vi "Halvorsen_1D_Lyapunov.vi"(11 "Initial Conditions":ext[](array[numeric])=[0.150000000000000000005, 0.1, 0.1]) -> ()   [LabVIEW 2016]
panel:
  in  "Initial Conditions Inc.":ext[](array[numeric])=[1e-8, 1e-8, 1e-8]
  in  "Tab Control":T1(tab)
  out "Mode Analysis":cluster{ext[], dbl[]}[](graph)=[{array[380 elements], [21.0, 25.0, 13.0, 26.0, 10.0, 21.0, 27.0, 22.0, 5.0, 15.0, 19.0, 19.0, 14.0, 15.0, 28.0, 21.0, 17.0, 26.0, 16.0, 16.0, 21.0, 21.0, 18.0, 1.0, 10.0, 13.0, 12.0, 14.0, 13.0, 12.0, 10.0, 16.0, 1.0, 10.0, 2.0, 16.0, 21.0, 4.0, 24.0, 20.0, 18.0, 14.0, 8.0, 23.0, 20.0, 11.0, 16.0, 26.0, 23.0, 25.0, 7.0, 16.0, 14.0, 17.0, 23.0, 13.0, 6.0, 21.0, 27.0, 24.0, 9.0, 7.0, 11.0, 19.0, 10.0, 17.0, 14.0, 8.0, 12.0, 16.0, 19.0, 19.0, 20.0, 16.0, 17.0, 22.0, 16.0, 18.0, 21.0, 27.0, 19.0, 23.0, 22.0, 19.0, 18.0, 17.0, 18.0, 13.0, 23.0, 14.0, 14.0, 19.0, 15.0, 22.0, 6.0, 16.0, 25.0, 18.0, 23.0, 18.0, 24.0, 22.0, 22.0, 20.0, 23.0, 21.0, 21.0, 19.0, 29.0, 18.0, 22.0, 16.0, 11.0, 16.0, 18.0, 18.0, 26.0, 24.0, 27.0, 28.0, 24.0, 21.0, 15.0, 24.0, 18.0, 19.0, 18.0, 23.0, 12.0, 20.0, 14.0, 17.0, 21.0, 24.0, 27.0, 27.0, 23.0, 19.0, 7.0, 24.0, 15.0, 24.0, 27.0, 19.0, 21.0, 21.0, 20.0, 16.0, 26.0, 21.0, 24.0, 24.0, 30.0, 19.0, 10.0, 18.0, 23.0, 25.0, 25.0, 20.0, 21.0, 21.0, 19.0, 24.0, 14.0, 18.0, 16.0, 21.0, 22.0, 20.0, 16.0, 24.0, 21.0, 24.0, 20.0, 20.0, 20.0, 24.0, 21.0, 22.0, 18.0, 27.0, 18.0, 21.0, 21.0, 18.0, 22.0, 20.0, 21.0, 21.0, 22.0, 19.0, 19.0, 15.0, 19.0, 19.0, 21.0, 18.0, 10.0, 20.0, 21.0, 20.0, 20.0, 18.0, 13.0, 20.0, 23.0, 18.0, 20.0, 17.0, 21.0, 20.0, 8.0, 5.0, 5.0, 19.0, 5.0, 16.0, 15.0, 5.0, 13.0, 19.0, 17.0, 17.0, 19.0, 13.0, 18.0, 19.0, 19.0, 20.0, 17.0, 16.0, 14.0, 16.0, 17.0, 15.0, 14.0, 15.0, 8.0, 17.0, 4.0, 17.0, 15.0, 17.0, 17.0, 16.0, 20.0, 17.0, 11.0, 7.0, 6.0, 11.0, 18.0, 8.0, 8.0, 18.0, 9.0, 16.0, 16.0, 19.0, 18.0, 15.0, 17.0, 16.0, 13.0, 13.0, 6.0, 5.0, 5.0, 4.0, 4.0, 4.0, 6.0, 19.0, 17.0, 8.0, 14.0, 15.0, 14.0, 17.0, 17.0, 10.0, 18.0, 11.0, 17.0, 12.0, 17.0, 2.0, 2.0, 1.0, 1.0, 2.0, 2.0, 2.0, 2.0, 2.0, 2.0, 2.0, 2.0, 2.0, 2.0, 2.0, 2.0, 2.0, 2.0, 2.0, 2.0, 4.0, 2.0, 17.0, 5.0, 4.0, 5.0, 8.0, 10.0, 12.0, 13.0, 13.0, 11.0, 9.0, 7.0, 2.0, 2.0, 2.0, 2.0, 2.0, 2.0, 2.0, 2.0, 2.0, 1.0, 2.0, 2.0, 2.0, 2.0, 2.0, 2.0, 2.0, 2.0, 2.0, 2.0, 2.0, 2.0, 2.0, 2.0, 2.0, 2.0, 2.0, 2.0, 2.0, 2.0, 1.0, 2.0, 5.0, 15.0, 12.0, 22.0, 13.0, 13.0, 9.0, 18.0, 10.0, 19.0, 17.0, 23.0, 23.0, 9.0, 7.0, 18.0, 21.0, 20.0, 19.0, 20.0, 20.0, 20.0, 9.0, 19.0, 18.0, 23.0, 17.0]}, {array[380 elements], [22.0, 26.0, 14.0, 26.0, 11.0, 21.0, 28.0, 23.0, 6.0, 16.0, 20.0, 20.0, 15.0, 16.0, 29.0, 21.0, 17.0, 26.0, 17.0, 17.0, 22.0, 22.0, 19.0, 1.0, 11.0, 14.0, 12.0, 15.0, 14.0, 13.0, 11.0, 17.0, 0.0, 10.0, 3.0, 17.0, 22.0, 5.0, 24.0, 20.0, 19.0, 15.0, 9.0, 23.0, 21.0, 12.0, 16.0, 27.0, 24.0, 25.0, 7.0, 17.0, 15.0, 18.0, 24.0, 14.0, 7.0, 22.0, 25.0, 25.0, 10.0, 8.0, 12.0, 20.0, 11.0, 17.0, 15.0, 8.0, 13.0, 17.0, 19.0, 19.0, 21.0, 17.0, 18.0, 22.0, 17.0, 18.0, 19.0, 26.0, 17.0, 23.0, 22.0, 19.0, 18.0, 17.0, 18.0, 13.0, 24.0, 14.0, 10.0, 20.0, 16.0, 22.0, 7.0, 17.0, 24.0, 13.0, 21.0, 17.0, 24.0, 19.0, 21.0, 20.0, 22.0, 21.0, 21.0, 20.0, 30.0, 19.0, 20.0, 16.0, 10.0, 15.0, 16.0, 18.0, 24.0, 24.0, 25.0, 27.0, 24.0, 22.0, 16.0, 25.0, 18.0, 20.0, 18.0, 23.0, 12.0, 20.0, 15.0, 9.0, 21.0, 24.0, 25.0, 25.0, 22.0, 17.0, 5.0, 25.0, 15.0, 23.0, 26.0, 18.0, 22.0, 21.0, 20.0, 15.0, 26.0, 19.0, 22.0, 25.0, 27.0, 19.0, 10.0, 18.0, 24.0, 26.0, 22.0, 20.0, 21.0, 21.0, 18.0, 24.0, 13.0, 19.0, 15.0, 21.0, 22.0, 16.0, 17.0, 22.0, 22.0, 22.0, 19.0, 19.0, 19.0, 19.0, 21.0, 23.0, 18.0, 26.0, 19.0, 20.0, 21.0, 18.0, 18.0, 21.0, 19.0, 21.0, 20.0, 16.0, 18.0, 13.0, 13.0, 19.0, 21.0, 14.0, 5.0, 19.0, 21.0, 20.0, 19.0, 19.0, 8.0, 19.0, 20.0, 17.0, 20.0, 14.0, 18.0, 17.0, 6.0, 5.0, 6.0, 18.0, 5.0, 15.0, 10.0, 4.0, 10.0, 16.0, 16.0, 17.0, 19.0, 14.0, 19.0, 18.0, 19.0, 18.0, 15.0, 13.0, 12.0, 17.0, 16.0, 15.0, 13.0, 12.0, 7.0, 18.0, 4.0, 15.0, 16.0, 14.0, 17.0, 16.0, 19.0, 12.0, 7.0, 6.0, 4.0, 6.0, 16.0, 8.0, 7.0, 19.0, 8.0, 14.0, 17.0, 16.0, 19.0, 13.0, 17.0, 13.0, 11.0, 12.0, 5.0, 4.0, 4.0, 4.0, 4.0, 4.0, 4.0, 19.0, 17.0, 8.0, 13.0, 14.0, 10.0, 16.0, 14.0, 11.0, 15.0, 11.0, 14.0, 13.0, 15.0, 2.0, 2.0, 1.0, 1.0, 2.0, 2.0, 2.0, 2.0, 2.0, 2.0, 2.0, 2.0, 2.0, 2.0, 2.0, 2.0, 2.0, 2.0, 2.0, 2.0, 2.0, 2.0, 9.0, 4.0, 4.0, 4.0, 4.0, 4.0, 4.0, 4.0, 3.0, 2.0, 2.0, 2.0, 2.0, 2.0, 2.0, 2.0, 2.0, 2.0, 2.0, 2.0, 2.0, 1.0, 2.0, 2.0, 2.0, 2.0, 2.0, 2.0, 2.0, 2.0, 2.0, 2.0, 2.0, 2.0, 2.0, 2.0, 2.0, 2.0, 2.0, 2.0, 2.0, 2.0, 1.0, 2.0, 2.0, 15.0, 10.0, 15.0, 12.0, 10.0, 8.0, 12.0, 9.0, 14.0, 13.0, 14.0, 13.0, 6.0, 6.0, 12.0, 12.0, 14.0, 16.0, 15.0, 15.0, 13.0, 8.0, 15.0, 13.0, 16.0, 11.0]}]
  out "Waveform Graph":ext[][](graph)
  out "?":cluster{ext[], ext[]}[](graph)
  out "Bifurcation Diagram":cluster{ext[], ext[]}(graph)
  in  "Parameter Index":i32
  in  "Final Parameter Value":dbl=0.2
  in  "Param_Inc":dbl[](array[numeric])=[0.0005, 0.0, 0.0]
  in  "Initial_Parameter_Vector":ext[](array[numeric])=[0.01, 0.1, 0.1]
  out "Current_Param":ext[](array[numeric])=[0.20000000000000000395, 0.1, 0.1]
  in  "Variable":u16(ring) items=["x", "y", "z"]
  in  "Время, с":ext=500.0
  in  "Hmin":ext=0.00099999999999999999996
  in  "Hmax":ext=1.0
  in  "tolerance":ext=1e-13
  in  "Шаг h, с":ext=0.01
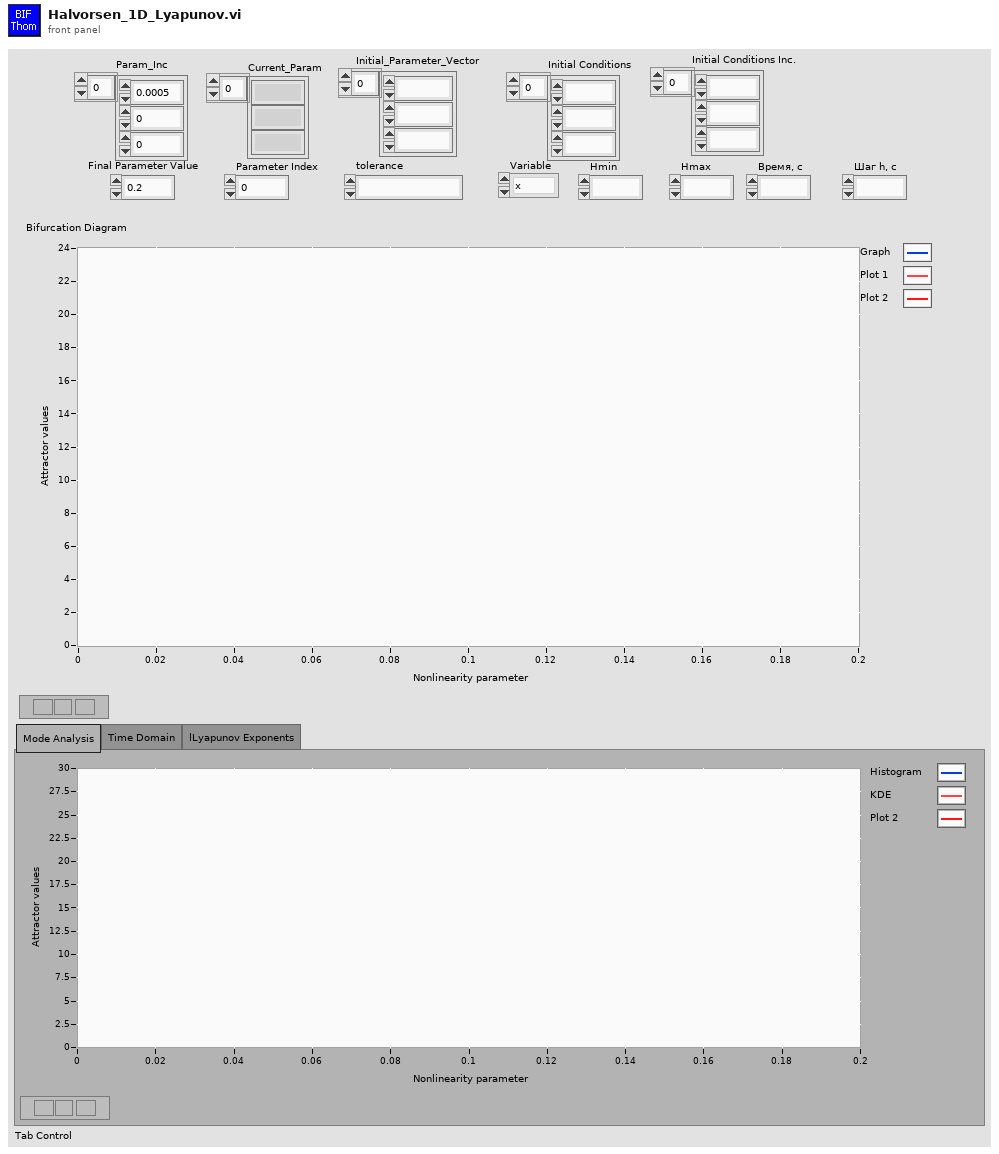
[diagram p1: front panel]
types:
  T1 = enum32{"Mode Analysis", "Time Domain", "lLyapunov Exponents"}
  T2 = enum16{"Euler", "Cromer 1", "Cromer 2", "D1", "D2", "PD1", "PD2", "CD1", "CD2", "CD3", "CD4", "IMP", "LIMP", "IEuler", "SEMP", "SIMP", "EMP", "MEMP"}
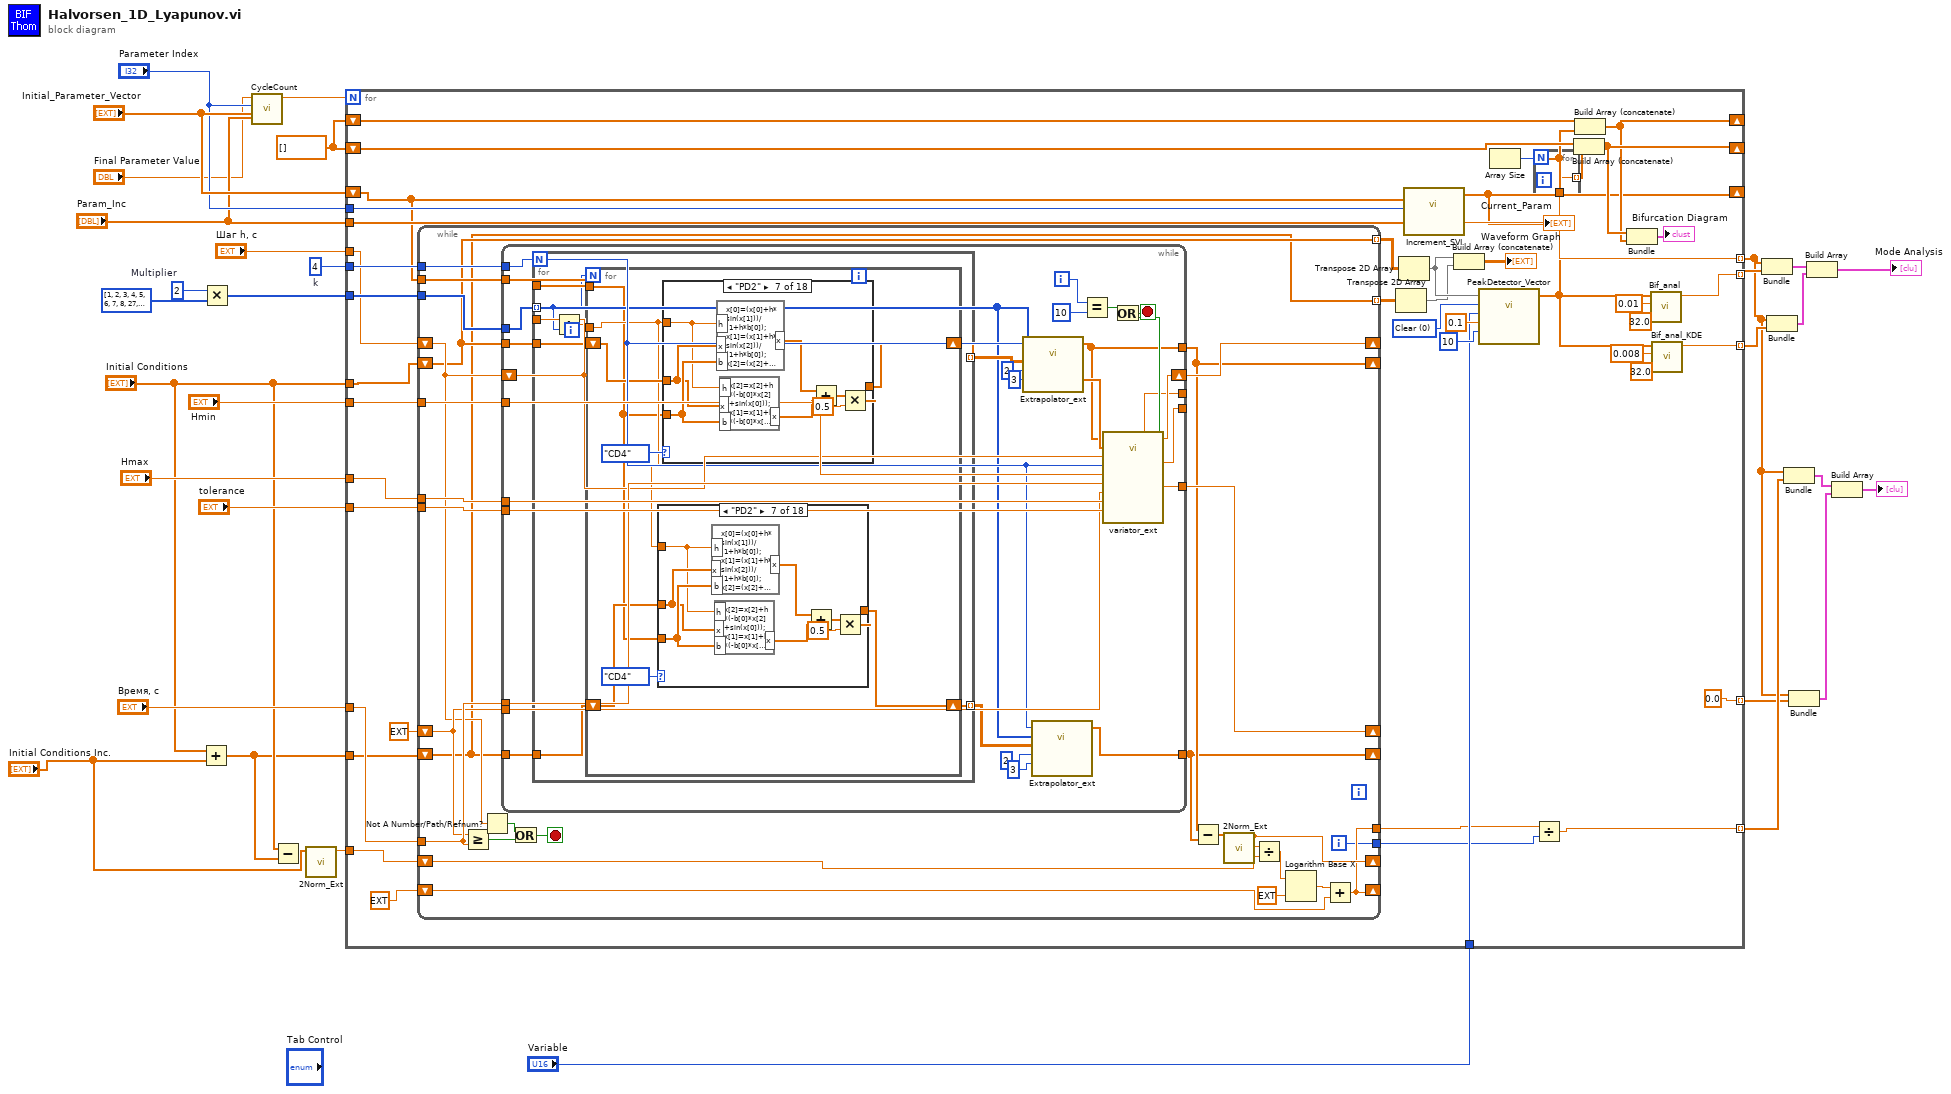
[diagram p0: block diagram]
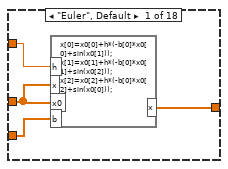
[diagram p2: hidden frame]
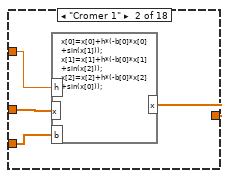
[diagram p3: hidden frame]
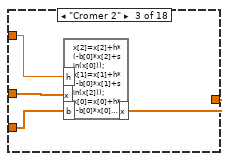
[diagram p4: hidden frame]
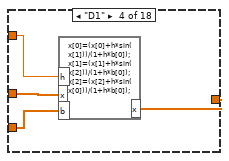
[diagram p5: hidden frame]
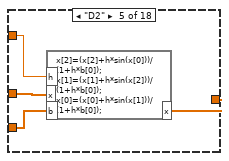
[diagram p6: hidden frame]
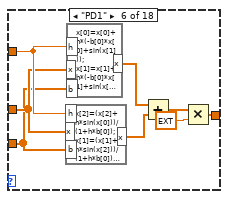
[diagram p7: hidden frame]
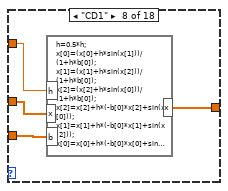
[diagram p8: hidden frame]
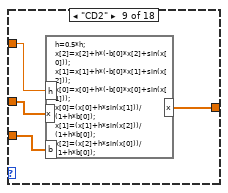
[diagram p9: hidden frame]
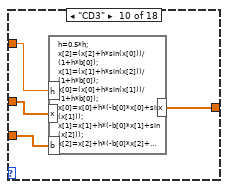
[diagram p10: hidden frame]
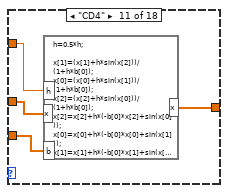
[diagram p11: hidden frame]
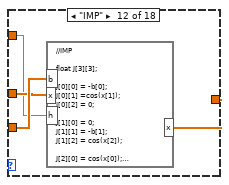
[diagram p12: hidden frame]
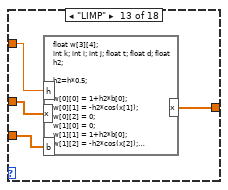
[diagram p13: hidden frame]
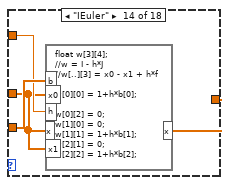
[diagram p14: hidden frame]
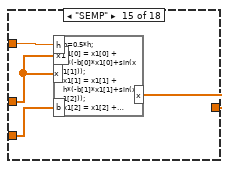
[diagram p15: hidden frame]
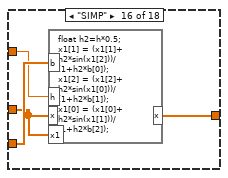
[diagram p16: hidden frame]
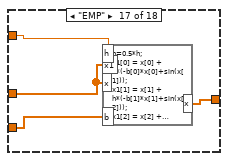
[diagram p17: hidden frame]
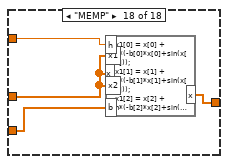
[diagram p18: hidden frame]
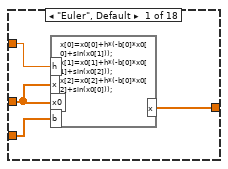
[diagram p19: hidden frame]
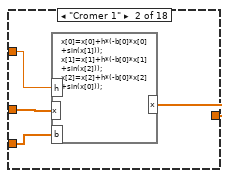
[diagram p20: hidden frame]
diagram:
  w16 = ext[] []
  w18 = 4  # k
  w21 = 2  # Multiplier
  n1 = Add(x="Initial Conditions", y="Initial Conditions Inc.") -> (x+y=w9:ext[])
  n2 = Multiply(x=w21, y=i32[] [1, 2, 3, 4, 5, 6, 7, 8, 27, 30, 33] ("n")) -> (x*y=w19:i32[])
  n3 = call "CycleCount.vi"("Increment_Vector"="Param_Inc", "Parameter_Vector"="Initial_Parameter_Vector", "Parameter Number"="Parameter Index", "Final_Parameter_Value"="Final Parameter Value") -> ("Cycle Count"=w17:ext)  [unwired: 5 in, 2 out]
  n4 = Subtract(x="Initial Conditions", y=w9) -> ()  [unwired: 1 out]
  n5 = call "2Norm_Ext.vi"("Input vector"="Initial Conditions Inc.") -> ("2 Norm"=w8:ext)  [unwired: 10 in]
  n6 = for {
    N: w17 -> [_]
    tunnel: w18 -> [w52]
    tunnel: "Шаг h, с" -> [w43]
    tunnel: "Время, с" -> [w47]
    tunnel: "tolerance" -> [w45]
    tunnel: "Hmin" -> [w49]
    tunnel: "Hmax" -> [w48]
    tunnel: w19 -> [w44]
    tunnel: "Initial Conditions" -> [w50]
    shift-right: [w54] -> _
    shift-left: "Initial_Parameter_Vector" -> [w51]
    tunnel: "Parameter Index" -> [w72]
    tunnel: "Param_Inc" -> [w71]
    tunnel: [w70] -> w15 mode=indexing
    tunnel: "Variable" -> [w69]
    shift-right: [w62] -> _
    shift-left: w16 -> [w67]
    shift-right: [w63] -> _
    shift-left: w16 -> [w66]
    tunnel: [w61] -> w6 mode=indexing
    tunnel: [w55] -> w12 mode=indexing
    tunnel: w9 -> [w42]
    tunnel: w8 -> [w40]
    tunnel: [w34] -> w7 mode=indexing
    tunnel: [0.0] -> w5 mode=indexing
    w75 = u16 0 items=["Clear", "Absolute", "Positive"] ("Signal Mode")
    n7 = while {
      shift-right: [w82] -> _
      shift-left: w50 -> [w88]
      tunnel: w44 -> [w102]
      tunnel: w52 -> [w101]
      shift-right: [w97] -> _
      shift-left: w43 -> [w90]
      shift-right: [w94] -> _
      shift-left: ext 0.0 ("New time") -> [w95]
      tunnel: w47 -> [w96]
      tunnel: w45 -> [w98]
      tunnel: w49 -> [w100]
      tunnel: w48 -> [w99]
      tunnel: w51 -> [w93]
      tunnel: [w88] -> w53 mode=indexing
      shift-right: [w81] -> _
      shift-left: w42 -> [w78]
      shift-right: [w79] -> _
      shift-left: w40 -> [w83]
      shift-right: [w77] -> _
      shift-left: ext 0.0 -> [w84]
      tunnel: [w78] -> w39 mode=indexing
      tunnel: [w77] -> w33
      tunnel: [w76] -> w32
      i -> [w76]
      stop <- w92 stop-if-true
      n8 = Greater Or Equal?(x=w95, y=w96) -> (x >= y?=w91:bool)
      n9 = Not A Number/Path/Refnum?(number/path/refnum=w90) -> (NaN/Path/Refnum?=w89:bool)
      n10 = while {
        tunnel: w100 -> [w125]
        tunnel: w99 -> [w128]
        tunnel: w98 -> [w124]
        tunnel: w101 -> [w108]
        tunnel: w102 -> [w107]
        tunnel: w88 -> [w126]
        shift-right: [w119] -> w97
        shift-left: w90 -> [w111]
        tunnel: [w111] -> _
        tunnel: [w118] -> _
        tunnel: [w117] -> w82
        tunnel: w96 -> [w116]
        tunnel: w95 -> [w115]
        tunnel: [w113] -> w94
        tunnel: w93 -> [w112]
        tunnel: w78 -> [w109]
        tunnel: [w103] -> w81
        i -> [w114]
        stop <- w120 stop-if-true
        n11 = for {
          N: w108 -> [_]
          tunnel: w107 -> [w133] mode=indexing
          tunnel: w111 -> [w138]
          tunnel: w126 -> [w136]
          tunnel: [w137] -> w127 mode=indexing
          tunnel: w112 -> [w134]
          tunnel: w109 -> [w132]
          tunnel: [w131] -> w106 mode=indexing
          n12 = Divide(x=w138, y=w133) -> (x/y=w135:ext)
          n13 = for {
            N: w133 -> [_]
            shift-right: [w146] -> w137
            shift-left: w136 -> [w145]
            tunnel: w135 -> [w142]
            tunnel: w134 -> [w139]
            shift-right: [w140] -> w131
            shift-left: w132 -> [w141]
            n14 = case shown="\"PD2\"" T2."CD4" ("Method") {
              tunnel: w142 -> [w148 w154 w157 w161 w166 w169 w175 w185 w189 w194 w197 w199 w206 w209 w213 w216 w220 w224]
              tunnel: w139 -> [w150 w152 w155 w159 w164 w167 w177 w183 w187 w192 w195 w201 w203 w210 w211 w217 w221 w225]
              tunnel: w141 -> [w149 w153 w156 w160 w165 w168 w176 w184 w188 w193 w196 w200 w204 w208 w212 w215 w219 w226]
              tunnel: [w147 w151 w158 w162 w163 w170 w178 w186 w190 w191 w198 w202 w205 w207 w214 w218 w222 w223] -> w140
              frame "Euler", Default {
                n15 = formula code="x[0]=x0[0]+h*(-b[0]*x0[0]+sin(x0[1]));\nx[1]=x0[1]+h*(-b[0]*x0[1]+sin(x0[2]));\nx[2]=x0[2]+h*(-b[0]*x0[2]+sin(x0[0]));"("x"=w149, "x0"=w149, "b"=w150, "h"=w148) -> ("x"=w147:ext[])
              }
              frame "Cromer 1" {
                n16 = formula code="x[0]=x[0]+h*(-b[0]*x[0]+sin(x[1]));\nx[1]=x[1]+h*(-b[0]*x[1]+sin(x[2]));\nx[2]=x[2]+h*(-b[0]*x[2]+sin(x[0]));"("x"=w153, "b"=w152, "h"=w154) -> ("x"=w151:ext[])
              }
              frame "Cromer 2" {
                n17 = formula code="x[2]=x[2]+h*(-b[0]*x[2]+sin(x[0]));\nx[1]=x[1]+h*(-b[0]*x[1]+sin(x[2]));\nx[0]=x[0]+h*(-b[0]*x[0]+sin(x[1]));"("x"=w156, "b"=w155, "h"=w157) -> ("x"=w158:ext[])
              }
              frame "D1" {
                n18 = formula code="x[0]=(x[0]+h*sin(x[1]))/(1+h*b[0]);\nx[1]=(x[1]+h*sin(x[2]))/(1+h*b[0]);\nx[2]=(x[2]+h*sin(x[0]))/(1+h*b[0]);"("x"=w160, "b"=w159, "h"=w161) -> ("x"=w162:ext[])
              }
              frame "D2" {
                n19 = formula code="x[2]=(x[2]+h*sin(x[0]))/(1+h*b[0]);\nx[1]=(x[1]+h*sin(x[2]))/(1+h*b[0]);\nx[0]=(x[0]+h*sin(x[1]))/(1+h*b[0]);"("x"=w165, "b"=w164, "h"=w166) -> ("x"=w163:ext[])
              }
              frame "PD1" {
                n20 = formula code="x[2]=(x[2]+h*sin(x[0]))/(1+h*b[0]);\nx[1]=(x[1]+h*sin(x[2]))/(1+h*b[0]);\nx[0]=(x[0]+h*sin(x[1]))/(1+h*b[0]);"("x"=w168, "b"=w167, "h"=w169) -> ("x"=w172:ext[])
                n21 = formula code="x[0]=x[0]+h*(-b[0]*x[0]+sin(x[1]));\nx[1]=x[1]+h*(-b[0]*x[1]+sin(x[2]));\nx[2]=x[2]+h*(-b[0]*x[2]+sin(x[0]));"("x"=w168, "b"=w167, "h"=w169) -> ("x"=w171:ext[])
                n22 = Add(x=w171, y=w172) -> (x+y=w173:ext[])
                n23 = Multiply(x=w173, y=ext 0.5) -> (x*y=w170:ext[])
              }
              frame "PD2" {
                n24 = formula code="x[0]=(x[0]+h*sin(x[1]))/(1+h*b[0]);\nx[1]=(x[1]+h*sin(x[2]))/(1+h*b[0]);\nx[2]=(x[2]+h*sin(x[0]))/(1+h*b[0]);"("x"=w176, "b"=w177, "h"=w175) -> ("x"=w182:ext[])
                n25 = formula code="x[2]=x[2]+h*(-b[0]*x[2]+sin(x[0]));\nx[1]=x[1]+h*(-b[0]*x[1]+sin(x[2]));\nx[0]=x[0]+h*(-b[0]*x[0]+sin(x[1]));"("x"=w176, "b"=w177, "h"=w175) -> ("x"=w181:ext[])
                n26 = Add(x=w182, y=w181) -> (x+y=w180:ext[])
                n27 = Multiply(x=w180, y=0.5) -> (x*y=w178:ext[])
              }
              frame "CD1" {
                n28 = formula code="h=0.5*h;\nx[0]=(x[0]+h*sin(x[1]))/(1+h*b[0]);\nx[1]=(x[1]+h*sin(x[2]))/(1+h*b[0]);\nx[2]=(x[2]+h*sin(x[0]))/(1+h*b[0]);\nx[2]=x[2]+h*(-b[0]*x[2]+sin(x[0]));\nx[1]=x[1]+h*(-b[0]*x[1]+sin(x[2]));\nx[0]=x[0]+h*(-b[0]*x[0]+sin(x[1]));"("x"=w184, "b"=w183, "h"=w185) -> ("x"=w186:ext[])
              }
              frame "CD2" {
                n29 = formula code="h=0.5*h;\nx[2]=x[2]+h*(-b[0]*x[2]+sin(x[0]));\nx[1]=x[1]+h*(-b[0]*x[1]+sin(x[2]));\nx[0]=x[0]+h*(-b[0]*x[0]+sin(x[1]));\nx[0]=(x[0]+h*sin(x[1]))/(1+h*b[0]);\nx[1]=(x[1]+h*sin(x[2]))/(1+h*b[0]);\nx[2]=(x[2]+h*sin(x[0]))/(1+h*b[0]);"("x"=w188, "b"=w187, "h"=w189) -> ("x"=w190:ext[])
              }
              frame "CD3" {
                n30 = formula code="h=0.5*h;\nx[2]=(x[2]+h*sin(x[0]))/(1+h*b[0]);\nx[1]=(x[1]+h*sin(x[2]))/(1+h*b[0]);\nx[0]=(x[0]+h*sin(x[1]))/(1+h*b[0]);\nx[0]=x[0]+h*(-b[0]*x[0]+sin(x[1]));\nx[1]=x[1]+h*(-b[0]*x[1]+sin(x[2]));\nx[2]=x[2]+h*(-b[0]*x[2]+sin(x[0]));"("x"=w193, "b"=w192, "h"=w194) -> ("x"=w191:ext[])
              }
              frame "CD4" {
                n31 = formula code="h=0.5*h;\n\nx[1]=(x[1]+h*sin(x[2]))/(1+h*b[0]);\nx[0]=(x[0]+h*sin(x[1]))/(1+h*b[0]);\nx[2]=(x[2]+h*sin(x[0]))/(1+h*b[0]);\nx[2]=x[2]+h*(-b[0]*x[2]+sin(x[0]));\nx[0]=x[0]+h*(-b[0]*x[0]+sin(x[1]));\nx[1]=x[1]+h*(-b[0]*x[1]+sin(x[2]));"("x"=w196, "b"=w195, "h"=w197) -> ("x"=w198:ext[])
              }
              frame "IMP" {
                n32 = formula code="//IMP\n\nfloat J[3][3];\n\nJ[0][0] = -b[0]; \nJ[0][1] =cos(x[1]); \nJ[0][2] = 0; \n\nJ[1][0] = 0; \nJ[1][1] = -b[1];\nJ[1][2] = cos(x[2]);\n\nJ[2][0] = cos(x[0]); \nJ[2][1] =0;\nJ[2][2] = -b[2];\n\n\nfloat w[3][4], Z[3], a[3], Zn[3], dz;\nfloat tol;\nint k; int i; int j; float t; float d;\ntol = 1e-14;\nint nnewtmax = 3, nnewt;\ndz = 2e-13;\nnnewt = 0;\n\nZ[0] = x[0]; Z[1] = x[1]; Z[2] = x[2];\nwhile ( (dz > tol) && (nnewt < nnewtmax)){\n\nfor(i=0;i<3;i++){\nfor(j=0;j<3;j++){\nif (i==j)\nw[i][j]=1 - 0.5*h*J[i][j];\nelse\nw[i][j]= - 0.5*h*J[i][j];\n}}\n\n\n\na[0] = 0.5*(x[0] + Z[0]);\na[1] = 0.5*(x[1] + Z[1]);\na[2] = 0.5*(x[2] + Z[2]);\n\n\n\nw[0][3]=-Z[0]+x[0]+h*(-b[0]*a[0]+sin(a[1]));\nw[1][3]= -Z[1]+x[1]+h*(-b[1]*a[1]+sin(a[2]));\nw[2][3]= -Z[2]+x[2]+h*(-b[2]*a[2]+sin(a[0]));\n\n\nfor(k = 0; k <= 1; k++){\n\tint l = k;\n\n\tfor( i = k+1; i<= 2; i++){\n\t\tif( abs(w[i][k]) > abs(w[l][k]) ){\n\t\t\tl = i;\n\t\t}\n\t}\n\tif (l != k){\n\t\tfor( j = 0; j <= 3; j++){\n\t\t\tif ((j == 0) || (j >= k)){\n\t\t\t\tt = w[k][j];\n\t\t\t\tw[k][j] = w[l][j];\n\t\t\t\tw[l][j] = t;\n\t\t\t}\n\t\t}\n\t}\t\n\n\td = 1.0 / w[k][k];\n\tfor( i=(k+1); i <=(2); i++){\n\t\tif (w[i][k] == 0){\n\t\t\tcontinue;\n\t\t}\n\t\tt = w[i][k] * d;\n\t\tfor ( j = k; j <= (3); j++) {\n\t\t\tif (w[k][j] != 0){\n\t\t\t\tw[i][j] = w[i][j] - t * w[k][j];\n\t\t\t}\n\t\t}\n\t}\n}\nfor( i=(3); i >= 2; i--){\n\tfor( j=1; j <= i-1; j++){\n\t\tt = w[i - j - 1][i - 1]/w[ i -1][i - 1];\n\t\tw[i-j - 1][ 3] = w[i-j -1][3] - t*w[i - 1][ 3];\n\t}\n\tw[i-1][ 3] = w[i - 1][3]/w[ i -1][i - 1];\n}\nw[0][3] = w[0][3]/w[0][0];\nZn[0] = Z[0]+ w[0][3];\nZn[1] = Z[1]+ w[1][3];\nZn[2] = Z[2]+ w[2][3];\n\ndz = ( (Zn[0] - Z[0])**2 + (Zn[1] - Z[1])**2 + (Zn[2] - Z[2])**2 )**0.5;\nZ[0] = Zn[0];\nZ[1] = Zn[1];\nZ[2] = Zn[2];\n\n\nnnewt ++;\n}\n\nx[0] = Zn[0];\nx[1] = Zn[1];\nx[2] = Zn[2];"("x"=w200, "h"=w199, "b"=w201) -> ("x"=w202:ext[])
              }
              frame "LIMP" {
                n33 = formula code="float w[3][4];\nint k; int i; int j; float t; float d; float h2;\n\nh2=h*0.5;\n\nw[0][0] = 1+h2*b[0];\nw[0][1] = -h2*cos(x[1]);\nw[0][2] = 0;\nw[1][0] = 0;\nw[1][1] = 1+h2*b[0];\nw[1][2] = -h2*cos(x[2]);\nw[2][0] = -h2*cos(x[0]);\nw[2][1] = 0;\nw[2][2] = 1+h2*b[0];\n\nw[0][3] = h*(-b[0]*x[0]+sin(x[1]));\nw[1][3] = h*(-b[0]*x[1]+sin(x[2]));\nw[2][3] = h*(-b[0]*x[2]+sin(x[0]));\n\nint HEIGHT = 3;\nint  WIDTH = 4;\nfor(k = 0; k <= HEIGHT-2; k++){\n\nint\tl = k;\n\nfor( i = k+1;  i<= HEIGHT-1; i++){\n\t\t\tif( abs(w[i][k]) > abs(w[l][k]) ){\n\t\t\t\tl = i;\n    }\n   }\n\t\tif (l != k){\n\t\t\tfor( j = 0; j <= WIDTH-1; j++){\n\t\t\t\tif ((j == 0) || (j >= k)){\n\t\t\t\t\tt = w[k][j];\n\t\t\t\t\tw[k][j] = w[l][j];\n\t\t\t\t\tw[l][j] = t;\n                }\n            }\n        }\n\n\t\td = 1.0 / w[k][k];\n\t\tfor( i=(k+1); i <=(HEIGHT-1); i++){\n\t\t\tif (w[i][k] == 0){\n                continue;\n            }\n\t\t\tt = w[i][k] * d;\n\t\t\tfor ( j = k; j <= (WIDTH-1); j++) {\n\t\t\t\tif (w[k][j] != 0){\n\t\t\t\t\tw[i][j] = w[i][j] - t * w[k][j];\n                }\n            }\n        }\n    }\n    \n\t\n    for( i=(HEIGHT); i >= 2; i--){ \n        for( j=1; j <= i-1; j++){\n            t = w[i - j - 1][i - 1]/w[ i -1][i - 1];\n            w[i-j - 1][ WIDTH- 1] = w[i-j -1][ WIDTH -1] - t*w[i - 1][ WIDTH -1];\n        }\n        w[i-1][ WIDTH-1] = w[i - 1][ WIDTH - 1]/w[ i -1][i - 1];\n    }\n    w[0][ WIDTH - 1] = w[0][ WIDTH -1]/w[0][0];\n\n    \n    x[0] =x[0]+ w[0][WIDTH - 1];\n    x[1] = x[1]+w[1][WIDTH - 1];\n    x[2] = x[2]+w[2][WIDTH - 1];"("x"=w204, "b"=w203, "h"=w206) -> ("x"=w205:ext[])
              }
              frame "IEuler" {
                n34 = formula code="float w[3][4];\n//w = I - h*J\n//w[..][3] = x0 - x1 + h*f\n\nw[0][0] = 1+h*b[0];\n\nw[0][2] = 0;\nw[1][0] = 0;\nw[1][1] = 1+h*b[1];\nw[2][1] = 0;\nw[2][2] = 1+h*b[2];\n\n\n\nfloat tol = 1e-12;\nfloat dx = 2*tol;\n\nint nmax = 10;\nint n = 0;\n//цикл по Ньютонам\nwhile ((dx > tol)&&(n < nmax)){\n\nw[0][1] = -h*cos(x[1]);\nw[1][2] = -h*cos(x[2]);\nw[2][0] = -h*cos(x[0]);\n\nw[0][3] = x0[0] - x1[0] +  h*(-b[0]*x[0]+sin(x[1]));\nw[1][3] = x0[1] - x1[1] + h*(-b[1]*x[1]+sin(x[2]));\nw[2][3] = x0[2] - x1[2] + h*(-b[2]*x[2]+sin(x[0]));\n\nint HEIGHT = 3;\nint  WIDTH = 4;\nint k; int i; int j; float t; float d;\n\nfor(k = 0; k <= HEIGHT-2; k++){\n\tint\tl = k;\n\tfor( i = k+1;  i<= HEIGHT-1; i++){\n\t\t\t\tif( abs(w[i][k]) > abs(w[l][k]) ){\n\t\t\t\t\tl = i;\n\t\t}\n   }\n\t\tif (l != k){\n\t\t\tfor( j = 0; j <= WIDTH-1; j++){\n\t\t\t\tif ((j == 0) || (j >= k)){\n\t\t\t\t\tt = w[k][j];\n\t\t\t\t\tw[k][j] = w[l][j];\n\t\t\t\t\tw[l][j] = t;\n                }\n            }\n        }\n\t\t\n\t\td = 1.0 / w[k][k];\n\t\tfor( i=(k+1); i <=(HEIGHT-1); i++){\n\t\t\tif (w[i][k] == 0){\n                continue;\n            }\n\t\t\tt = w[i][k] * d;\n\t\t\tfor ( j = k; j <= (WIDTH-1); j++) {\n\t\t\t\tif (w[k][j] != 0){\n\t\t\t\t\tw[i][j] = w[i][j] - t * w[k][j];\n                }\n            }\n        }\n    }\n\n    for( i=(HEIGHT); i >= 2; i--){ \n        for( j=1; j <= i-1; j++){\n            t = w[i - j - 1][i - 1]/w[ i -1][i - 1];\n            w[i-j - 1][ WIDTH- 1] = w[i-j -1][ WIDTH -1] - t*w[i - 1][ WIDTH -1];\n        }\n        w[i-1][ WIDTH-1] = w[i - 1][ WIDTH - 1]/w[ i -1][i - 1];\n    }\n    w[0][ WIDTH - 1] = w[0][ WIDTH -1]/w[0][0];\n\n    \n    x1[0] =x[0]+ w[0][WIDTH - 1];\n    x1[1] = x[1]+w[1][WIDTH - 1];\n    x1[2] = x[2]+w[2][WIDTH - 1];\n\ndx = sqrt((x1[0] - x[0])**2 + (x1[1] - x[1])**2 + (x1[2] - x[2])**2);\nn++;\n\nx[0] = x1[0]; x[1] = x1[1]; x[2] = x1[2];\n\n}"("x"=w208, "h"=w209, "x1"=w208, "b"=w210, "x0"=w208) -> ("x"=w207:ext[])
              }
              frame "SEMP" {
                n35 = formula code="h=0.5*h;\nx1[0] = x1[0] + h*(-b[0]*x1[0]+sin(x1[1])); \nx1[1] = x1[1] + h*(-b[1]*x1[1]+sin(x1[2])); \nx1[2] = x1[2] + h*(-b[2]*x1[2]+sin(x1[0]));\n\nx[0] = x[0] + h*(-b[0]*x1[0]+sin(x1[1])); \nx[1] = x[1] + h*(-b[1]*x1[1]+sin(x1[2])); \nx[2] = x[2] + h*(-b[2]*x1[2]+sin(x1[0]));"("x"=w212, "x1"=w212, "h"=w213, "b"=w211) -> ("x"=w214:ext[])
              }
              frame "SIMP" {
                n36 = formula code="float h2=h*0.5;\nx1[1] = (x1[1]+ h2*sin(x1[2]))/(1+h2*b[0]);\nx1[2] = (x1[2]+ h2*sin(x1[0]))/(1+h2*b[1]);\nx1[0] = (x1[0]+ h2*sin(x1[1]))/(1+h2*b[2]);\n\n\nx[0] = x[0] + h*(-b[0]*x1[0]+sin(x1[1]));\nx[1] = x[1] + h*(-b[1]*x1[1]+sin(x1[2]));\nx[2] = x[2] + h*(-b[2]*x1[2]+sin(x1[0]));"("x"=w215, "h"=w216, "x1"=w215, "b"=w217) -> ("x"=w218:ext[])
              }
              frame "EMP" {
                n37 = formula code="h=0.5*h;\nx1[0] = x[0] + h*(-b[0]*x[0]+sin(x[1])); \nx1[1] = x[1] + h*(-b[1]*x[1]+sin(x[2])); \nx1[2] = x[2] + h*(-b[2]*x[2]+sin(x[0]));\n\nx[0] = x[0] + h*(-b[0]*x1[0]+sin(x1[1])); \nx[1] = x[1] + h*(-b[1]*x1[1]+sin(x1[2])); \nx[2] = x[2] + h*(-b[2]*x1[2]+sin(x1[0]));"("x"=w219, "x1"=w219, "h"=w220, "b"=w221) -> ("x"=w222:ext[])
              }
              frame "MEMP" {
                n38 = formula code="x1[0] = x[0] + h*(-b[0]*x[0]+sin(x[1])); \nx1[1] = x[1] + h*(-b[1]*x[1]+sin(x[2])); \nx1[2] = x[2] + h*(-b[2]*x[2]+sin(x[0]));\nh=2*h;\n\nx2[0] = x[0] + h*(-b[0]*x1[0]+sin(x1[1])); \nx2[1] = x[1] + h*(-b[1]*x1[1]+sin(x1[2])); \nx2[2] = x[2] + h*(-b[2]*x1[2]+sin(x1[0]));\n\nx[0]=x1[0];\nx[1]=x1[1];\nx[2]=x1[2];\nx1[0]=x2[0];\nx1[1]=x2[1];\nx1[2]=x2[2];\nh=h*0.5;\nx2[0]=(x[0]+x1[0]+h*(-b[0]*x1[0]+sin(x1[1])))/2;\nx2[1]=(x[1]+x1[1]+h*(-b[1]*x1[1]+sin(x1[2])))/2;\nx2[2]=(x[2]+x1[2]+h*(-b[2]*x1[2]+sin(x1[0])))/2;"("x"=w226, "x1"=w226, "h"=w224, "b"=w225, "x2"=w226) -> ("x"=w223:ext[])
              }
            }
            n39 = case shown="\"PD2\"" T2."CD4" ("Method") {
              tunnel: w142 -> [w228 w234 w237 w241 w246 w249 w255 w265 w269 w274 w277 w279 w286 w289 w293 w296 w300 w304]
              tunnel: w139 -> [w230 w232 w235 w239 w244 w247 w257 w263 w267 w272 w275 w281 w283 w290 w291 w297 w301 w305]
              tunnel: w145 -> [w229 w233 w236 w240 w245 w248 w256 w264 w268 w273 w276 w280 w284 w288 w292 w295 w299 w306]
              tunnel: [w227 w231 w238 w242 w243 w250 w258 w266 w270 w271 w278 w282 w285 w287 w294 w298 w302 w303] -> w146
              frame "Euler", Default {
                n40 = formula code="x[0]=x0[0]+h*(-b[0]*x0[0]+sin(x0[1]));\nx[1]=x0[1]+h*(-b[0]*x0[1]+sin(x0[2]));\nx[2]=x0[2]+h*(-b[0]*x0[2]+sin(x0[0]));"("x"=w229, "x0"=w229, "b"=w230, "h"=w228) -> ("x"=w227:ext[])
              }
              frame "Cromer 1" {
                n41 = formula code="x[0]=x[0]+h*(-b[0]*x[0]+sin(x[1]));\nx[1]=x[1]+h*(-b[0]*x[1]+sin(x[2]));\nx[2]=x[2]+h*(-b[0]*x[2]+sin(x[0]));"("x"=w233, "b"=w232, "h"=w234) -> ("x"=w231:ext[])
              }
              frame "Cromer 2" {
                n42 = formula code="x[2]=x[2]+h*(-b[0]*x[2]+sin(x[0]));\nx[1]=x[1]+h*(-b[0]*x[1]+sin(x[2]));\nx[0]=x[0]+h*(-b[0]*x[0]+sin(x[1]));"("x"=w236, "b"=w235, "h"=w237) -> ("x"=w238:ext[])
              }
              frame "D1" {
                n43 = formula code="x[0]=(x[0]+h*sin(x[1]))/(1+h*b[0]);\nx[1]=(x[1]+h*sin(x[2]))/(1+h*b[0]);\nx[2]=(x[2]+h*sin(x[0]))/(1+h*b[0]);"("x"=w240, "b"=w239, "h"=w241) -> ("x"=w242:ext[])
              }
              frame "D2" {
                n44 = formula code="x[2]=(x[2]+h*sin(x[0]))/(1+h*b[0]);\nx[1]=(x[1]+h*sin(x[2]))/(1+h*b[0]);\nx[0]=(x[0]+h*sin(x[1]))/(1+h*b[0]);"("x"=w245, "b"=w244, "h"=w246) -> ("x"=w243:ext[])
              }
              frame "PD1" {
                n45 = formula code="x[2]=(x[2]+h*sin(x[0]))/(1+h*b[0]);\nx[1]=(x[1]+h*sin(x[2]))/(1+h*b[0]);\nx[0]=(x[0]+h*sin(x[1]))/(1+h*b[0]);"("x"=w248, "b"=w247, "h"=w249) -> ("x"=w252:ext[])
                n46 = formula code="x[0]=x[0]+h*(-b[0]*x[0]+sin(x[1]));\nx[1]=x[1]+h*(-b[0]*x[1]+sin(x[2]));\nx[2]=x[2]+h*(-b[0]*x[2]+sin(x[0]));"("x"=w248, "b"=w247, "h"=w249) -> ("x"=w251:ext[])
                n47 = Add(x=w251, y=w252) -> (x+y=w253:ext[])
                n48 = Multiply(x=w253, y=ext 0.5) -> (x*y=w250:ext[])
              }
              frame "PD2" {
                n49 = formula code="x[0]=(x[0]+h*sin(x[1]))/(1+h*b[0]);\nx[1]=(x[1]+h*sin(x[2]))/(1+h*b[0]);\nx[2]=(x[2]+h*sin(x[0]))/(1+h*b[0]);"("x"=w256, "b"=w257, "h"=w255) -> ("x"=w262:ext[])
                n50 = formula code="x[2]=x[2]+h*(-b[0]*x[2]+sin(x[0]));\nx[1]=x[1]+h*(-b[0]*x[1]+sin(x[2]));\nx[0]=x[0]+h*(-b[0]*x[0]+sin(x[1]));"("x"=w256, "b"=w257, "h"=w255) -> ("x"=w261:ext[])
                n51 = Add(x=w262, y=w261) -> (x+y=w260:ext[])
                n52 = Multiply(x=w260, y=0.5) -> (x*y=w258:ext[])
              }
              frame "CD1" {
                n53 = formula code="h=0.5*h;\nx[0]=(x[0]+h*sin(x[1]))/(1+h*b[0]);\nx[1]=(x[1]+h*sin(x[2]))/(1+h*b[0]);\nx[2]=(x[2]+h*sin(x[0]))/(1+h*b[0]);\nx[2]=x[2]+h*(-b[0]*x[2]+sin(x[0]));\nx[1]=x[1]+h*(-b[0]*x[1]+sin(x[2]));\nx[0]=x[0]+h*(-b[0]*x[0]+sin(x[1]));"("x"=w264, "b"=w263, "h"=w265) -> ("x"=w266:ext[])
              }
              frame "CD2" {
                n54 = formula code="h=0.5*h;\nx[2]=x[2]+h*(-b[0]*x[2]+sin(x[0]));\nx[1]=x[1]+h*(-b[0]*x[1]+sin(x[2]));\nx[0]=x[0]+h*(-b[0]*x[0]+sin(x[1]));\nx[0]=(x[0]+h*sin(x[1]))/(1+h*b[0]);\nx[1]=(x[1]+h*sin(x[2]))/(1+h*b[0]);\nx[2]=(x[2]+h*sin(x[0]))/(1+h*b[0]);"("x"=w268, "b"=w267, "h"=w269) -> ("x"=w270:ext[])
              }
              frame "CD3" {
                n55 = formula code="h=0.5*h;\nx[2]=(x[2]+h*sin(x[0]))/(1+h*b[0]);\nx[1]=(x[1]+h*sin(x[2]))/(1+h*b[0]);\nx[0]=(x[0]+h*sin(x[1]))/(1+h*b[0]);\nx[0]=x[0]+h*(-b[0]*x[0]+sin(x[1]));\nx[1]=x[1]+h*(-b[0]*x[1]+sin(x[2]));\nx[2]=x[2]+h*(-b[0]*x[2]+sin(x[0]));"("x"=w273, "b"=w272, "h"=w274) -> ("x"=w271:ext[])
              }
              frame "CD4" {
                n56 = formula code="h=0.5*h;\n\nx[1]=(x[1]+h*sin(x[2]))/(1+h*b[0]);\nx[0]=(x[0]+h*sin(x[1]))/(1+h*b[0]);\nx[2]=(x[2]+h*sin(x[0]))/(1+h*b[0]);\nx[2]=x[2]+h*(-b[0]*x[2]+sin(x[0]));\nx[0]=x[0]+h*(-b[0]*x[0]+sin(x[1]));\nx[1]=x[1]+h*(-b[0]*x[1]+sin(x[2]));"("x"=w276, "b"=w275, "h"=w277) -> ("x"=w278:ext[])
              }
              frame "IMP" {
                n57 = formula code="//IMP\n\nfloat J[3][3];\n\nJ[0][0] = -b[0]; \nJ[0][1] =cos(x[1]); \nJ[0][2] = 0; \n\nJ[1][0] = 0; \nJ[1][1] = -b[1];\nJ[1][2] = cos(x[2]);\n\nJ[2][0] = cos(x[0]); \nJ[2][1] =0;\nJ[2][2] = -b[2];\n\n\nfloat w[3][4], Z[3], a[3], Zn[3], dz;\nfloat tol;\nint k; int i; int j; float t; float d;\ntol = 1e-14;\nint nnewtmax = 3, nnewt;\ndz = 2e-13;\nnnewt = 0;\n\nZ[0] = x[0]; Z[1] = x[1]; Z[2] = x[2];\nwhile ( (dz > tol) && (nnewt < nnewtmax)){\n\nfor(i=0;i<3;i++){\nfor(j=0;j<3;j++){\nif (i==j)\nw[i][j]=1 - 0.5*h*J[i][j];\nelse\nw[i][j]= - 0.5*h*J[i][j];\n}}\n\n\n\na[0] = 0.5*(x[0] + Z[0]);\na[1] = 0.5*(x[1] + Z[1]);\na[2] = 0.5*(x[2] + Z[2]);\n\n\n\nw[0][3]=-Z[0]+x[0]+h*(-b[0]*a[0]+sin(a[1]));\nw[1][3]= -Z[1]+x[1]+h*(-b[1]*a[1]+sin(a[2]));\nw[2][3]= -Z[2]+x[2]+h*(-b[2]*a[2]+sin(a[0]));\n\n\nfor(k = 0; k <= 1; k++){\n\tint l = k;\n\n\tfor( i = k+1; i<= 2; i++){\n\t\tif( abs(w[i][k]) > abs(w[l][k]) ){\n\t\t\tl = i;\n\t\t}\n\t}\n\tif (l != k){\n\t\tfor( j = 0; j <= 3; j++){\n\t\t\tif ((j == 0) || (j >= k)){\n\t\t\t\tt = w[k][j];\n\t\t\t\tw[k][j] = w[l][j];\n\t\t\t\tw[l][j] = t;\n\t\t\t}\n\t\t}\n\t}\t\n\n\td = 1.0 / w[k][k];\n\tfor( i=(k+1); i <=(2); i++){\n\t\tif (w[i][k] == 0){\n\t\t\tcontinue;\n\t\t}\n\t\tt = w[i][k] * d;\n\t\tfor ( j = k; j <= (3); j++) {\n\t\t\tif (w[k][j] != 0){\n\t\t\t\tw[i][j] = w[i][j] - t * w[k][j];\n\t\t\t}\n\t\t}\n\t}\n}\nfor( i=(3); i >= 2; i--){\n\tfor( j=1; j <= i-1; j++){\n\t\tt = w[i - j - 1][i - 1]/w[ i -1][i - 1];\n\t\tw[i-j - 1][ 3] = w[i-j -1][3] - t*w[i - 1][ 3];\n\t}\n\tw[i-1][ 3] = w[i - 1][3]/w[ i -1][i - 1];\n}\nw[0][3] = w[0][3]/w[0][0];\nZn[0] = Z[0]+ w[0][3];\nZn[1] = Z[1]+ w[1][3];\nZn[2] = Z[2]+ w[2][3];\n\ndz = ( (Zn[0] - Z[0])**2 + (Zn[1] - Z[1])**2 + (Zn[2] - Z[2])**2 )**0.5;\nZ[0] = Zn[0];\nZ[1] = Zn[1];\nZ[2] = Zn[2];\n\n\nnnewt ++;\n}\n\nx[0] = Zn[0];\nx[1] = Zn[1];\nx[2] = Zn[2];"("x"=w280, "h"=w279, "b"=w281) -> ("x"=w282:ext[])
              }
              frame "LIMP" {
                n58 = formula code="float w[3][4];\nint k; int i; int j; float t; float d; float h2;\n\nh2=h*0.5;\n\nw[0][0] = 1+h2*b[0];\nw[0][1] = -h2*cos(x[1]);\nw[0][2] = 0;\nw[1][0] = 0;\nw[1][1] = 1+h2*b[0];\nw[1][2] = -h2*cos(x[2]);\nw[2][0] = -h2*cos(x[0]);\nw[2][1] = 0;\nw[2][2] = 1+h2*b[0];\n\nw[0][3] = h*(-b[0]*x[0]+sin(x[1]));\nw[1][3] = h*(-b[0]*x[1]+sin(x[2]));\nw[2][3] = h*(-b[0]*x[2]+sin(x[0]));\n\nint HEIGHT = 3;\nint  WIDTH = 4;\nfor(k = 0; k <= HEIGHT-2; k++){\n\nint\tl = k;\n\nfor( i = k+1;  i<= HEIGHT-1; i++){\n\t\t\tif( abs(w[i][k]) > abs(w[l][k]) ){\n\t\t\t\tl = i;\n    }\n   }\n\t\tif (l != k){\n\t\t\tfor( j = 0; j <= WIDTH-1; j++){\n\t\t\t\tif ((j == 0) || (j >= k)){\n\t\t\t\t\tt = w[k][j];\n\t\t\t\t\tw[k][j] = w[l][j];\n\t\t\t\t\tw[l][j] = t;\n                }\n            }\n        }\n\n\t\td = 1.0 / w[k][k];\n\t\tfor( i=(k+1); i <=(HEIGHT-1); i++){\n\t\t\tif (w[i][k] == 0){\n                continue;\n            }\n\t\t\tt = w[i][k] * d;\n\t\t\tfor ( j = k; j <= (WIDTH-1); j++) {\n\t\t\t\tif (w[k][j] != 0){\n\t\t\t\t\tw[i][j] = w[i][j] - t * w[k][j];\n                }\n            }\n        }\n    }\n    \n\t\n    for( i=(HEIGHT); i >= 2; i--){ \n        for( j=1; j <= i-1; j++){\n            t = w[i - j - 1][i - 1]/w[ i -1][i - 1];\n            w[i-j - 1][ WIDTH- 1] = w[i-j -1][ WIDTH -1] - t*w[i - 1][ WIDTH -1];\n        }\n        w[i-1][ WIDTH-1] = w[i - 1][ WIDTH - 1]/w[ i -1][i - 1];\n    }\n    w[0][ WIDTH - 1] = w[0][ WIDTH -1]/w[0][0];\n\n    \n    x[0] =x[0]+ w[0][WIDTH - 1];\n    x[1] = x[1]+w[1][WIDTH - 1];\n    x[2] = x[2]+w[2][WIDTH - 1];"("x"=w284, "b"=w283, "h"=w286) -> ("x"=w285:ext[])
              }
              frame "IEuler" {
                n59 = formula code="float w[3][4];\n//w = I - h*J\n//w[..][3] = x0 - x1 + h*f\n\nw[0][0] = 1+h*b[0];\n\nw[0][2] = 0;\nw[1][0] = 0;\nw[1][1] = 1+h*b[1];\nw[2][1] = 0;\nw[2][2] = 1+h*b[2];\n\n\n\nfloat tol = 1e-12;\nfloat dx = 2*tol;\n\nint nmax = 10;\nint n = 0;\n//цикл по Ньютонам\nwhile ((dx > tol)&&(n < nmax)){\n\nw[0][1] = -h*cos(x[1]);\nw[1][2] = -h*cos(x[2]);\nw[2][0] = -h*cos(x[0]);\n\nw[0][3] = x0[0] - x1[0] +  h*(-b[0]*x[0]+sin(x[1]));\nw[1][3] = x0[1] - x1[1] + h*(-b[1]*x[1]+sin(x[2]));\nw[2][3] = x0[2] - x1[2] + h*(-b[2]*x[2]+sin(x[0]));\n\nint HEIGHT = 3;\nint  WIDTH = 4;\nint k; int i; int j; float t; float d;\n\nfor(k = 0; k <= HEIGHT-2; k++){\n\tint\tl = k;\n\tfor( i = k+1;  i<= HEIGHT-1; i++){\n\t\t\t\tif( abs(w[i][k]) > abs(w[l][k]) ){\n\t\t\t\t\tl = i;\n\t\t}\n   }\n\t\tif (l != k){\n\t\t\tfor( j = 0; j <= WIDTH-1; j++){\n\t\t\t\tif ((j == 0) || (j >= k)){\n\t\t\t\t\tt = w[k][j];\n\t\t\t\t\tw[k][j] = w[l][j];\n\t\t\t\t\tw[l][j] = t;\n                }\n            }\n        }\n\t\t\n\t\td = 1.0 / w[k][k];\n\t\tfor( i=(k+1); i <=(HEIGHT-1); i++){\n\t\t\tif (w[i][k] == 0){\n                continue;\n            }\n\t\t\tt = w[i][k] * d;\n\t\t\tfor ( j = k; j <= (WIDTH-1); j++) {\n\t\t\t\tif (w[k][j] != 0){\n\t\t\t\t\tw[i][j] = w[i][j] - t * w[k][j];\n                }\n            }\n        }\n    }\n\n    for( i=(HEIGHT); i >= 2; i--){ \n        for( j=1; j <= i-1; j++){\n            t = w[i - j - 1][i - 1]/w[ i -1][i - 1];\n            w[i-j - 1][ WIDTH- 1] = w[i-j -1][ WIDTH -1] - t*w[i - 1][ WIDTH -1];\n        }\n        w[i-1][ WIDTH-1] = w[i - 1][ WIDTH - 1]/w[ i -1][i - 1];\n    }\n    w[0][ WIDTH - 1] = w[0][ WIDTH -1]/w[0][0];\n\n    \n    x1[0] =x[0]+ w[0][WIDTH - 1];\n    x1[1] = x[1]+w[1][WIDTH - 1];\n    x1[2] = x[2]+w[2][WIDTH - 1];\n\ndx = sqrt((x1[0] - x[0])**2 + (x1[1] - x[1])**2 + (x1[2] - x[2])**2);\nn++;\n\nx[0] = x1[0]; x[1] = x1[1]; x[2] = x1[2];\n\n}"("x"=w288, "h"=w289, "x1"=w288, "b"=w290, "x0"=w288) -> ("x"=w287:ext[])
              }
              frame "SEMP" {
                n60 = formula code="h=0.5*h;\nx1[0] = x1[0] + h*(-b[0]*x1[0]+sin(x1[1])); \nx1[1] = x1[1] + h*(-b[1]*x1[1]+sin(x1[2])); \nx1[2] = x1[2] + h*(-b[2]*x1[2]+sin(x1[0]));\n\nx[0] = x[0] + h*(-b[0]*x1[0]+sin(x1[1])); \nx[1] = x[1] + h*(-b[1]*x1[1]+sin(x1[2])); \nx[2] = x[2] + h*(-b[2]*x1[2]+sin(x1[0]));"("x"=w292, "x1"=w292, "h"=w293, "b"=w291) -> ("x"=w294:ext[])
              }
              frame "SIMP" {
                n61 = formula code="float h2=h*0.5;\nx1[1] = (x1[1]+ h2*sin(x1[2]))/(1+h2*b[0]);\nx1[2] = (x1[2]+ h2*sin(x1[0]))/(1+h2*b[1]);\nx1[0] = (x1[0]+ h2*sin(x1[1]))/(1+h2*b[2]);\n\n\nx[0] = x[0] + h*(-b[0]*x1[0]+sin(x1[1]));\nx[1] = x[1] + h*(-b[1]*x1[1]+sin(x1[2]));\nx[2] = x[2] + h*(-b[2]*x1[2]+sin(x1[0]));"("x"=w295, "h"=w296, "x1"=w295, "b"=w297) -> ("x"=w298:ext[])
              }
              frame "EMP" {
                n62 = formula code="h=0.5*h;\nx1[0] = x[0] + h*(-b[0]*x[0]+sin(x[1])); \nx1[1] = x[1] + h*(-b[1]*x[1]+sin(x[2])); \nx1[2] = x[2] + h*(-b[2]*x[2]+sin(x[0]));\n\nx[0] = x[0] + h*(-b[0]*x1[0]+sin(x1[1])); \nx[1] = x[1] + h*(-b[1]*x1[1]+sin(x1[2])); \nx[2] = x[2] + h*(-b[2]*x1[2]+sin(x1[0]));"("x"=w299, "x1"=w299, "h"=w300, "b"=w301) -> ("x"=w302:ext[])
              }
              frame "MEMP" {
                n63 = formula code="x1[0] = x[0] + h*(-b[0]*x[0]+sin(x[1])); \nx1[1] = x[1] + h*(-b[1]*x[1]+sin(x[2])); \nx1[2] = x[2] + h*(-b[2]*x[2]+sin(x[0]));\nh=2*h;\n\nx2[0] = x[0] + h*(-b[0]*x1[0]+sin(x1[1])); \nx2[1] = x[1] + h*(-b[1]*x1[1]+sin(x1[2])); \nx2[2] = x[2] + h*(-b[2]*x1[2]+sin(x1[0]));\n\nx[0]=x1[0];\nx[1]=x1[1];\nx[2]=x1[2];\nx1[0]=x2[0];\nx1[1]=x2[1];\nx1[2]=x2[2];\nh=h*0.5;\nx2[0]=(x[0]+x1[0]+h*(-b[0]*x1[0]+sin(x1[1])))/2;\nx2[1]=(x[1]+x1[1]+h*(-b[1]*x1[1]+sin(x1[2])))/2;\nx2[2]=(x[2]+x1[2]+h*(-b[2]*x1[2]+sin(x1[0])))/2;"("x"=w306, "x1"=w306, "h"=w304, "b"=w305, "x2"=w306) -> ("x"=w303:ext[])
              }
            }
          }
        }
        n64 = call "Extrapolator_ext.vi"("Порядок экстраполятора"=2 ("Ext. Order"), "Dimension"=3 ("input variable"), "Х - нач. условия"=w127, "n"=w107, "k"=w108) -> ("TPrev"=w129:ext[], "Tout"=w117:ext[])  [unwired: 5 in]
        n65 = call "Extrapolator_ext.vi"("Порядок экстраполятора"=2 ("Ext. Order"), "Dimension"=3 ("input variable"), "Х - нач. условия"=w106, "n"=w107, "k"=w108) -> ("Tout"=w103:ext[])  [unwired: 5 in, 1 out]
        n66 = Equal?(x=w114, y=10) -> (x = y?=w122:bool)
        n67 = call "variator_ext.vi"("Tout"=w117, "tolerance"=w124, "Hmax"=w128, "TPrev"=w129, "Шаг h, с"=w111, "Current time"=w115, "k"=w108, "Hmin"=w125, "tmax"=w116) -> ("Hnew"=w119:ext, "error estimation"=w118:ext, "New time"=w113:ext, "stop"=w121:bool)  [unwired: 3 in]
        n68 = Or(x=w122, y=w121) -> (x .or. y?=w120:bool)
      }
      n69 = Or(x=w89, y=w91) -> (x .or. y?=w92:bool)
      n70 = Subtract(x=w82, y=w81) -> (x-y=w80:ext[])
      n71 = call "2Norm_Ext.vi"("Input vector"=w80) -> ("2 Norm"=w79:ext)  [unwired: 10 in]
      n72 = Divide(x=w79, y=w83) -> (x/y=w87:ext)
      n73 = Logarithm Base X(1:ext 10.0 ("x"), 2:w87) -> (0:w86:ext)
      n74 = Add(x=w86, y=w84) -> (x+y=w77:ext)
    }
    n75 = Transpose 2D Array(2D array=w39) -> (transposed array=w37:ext[][])
    n76 = Transpose 2D Array(2D array=w53) -> (transposed array=w38:ext[][])
    n77 = call "Increment_SVI.vi"("Increment_Vector"=w71, "Param_Index"=w72, "Parameter_Vector"=w51) -> ("Current_Parameter"=w61:ext, "Parameters_Out"=w54:ext[])  [unwired: 7 in]
    "Current_Param" <- w54
    n78 = Build Array (concatenate)(w38, w37) -> (→"Waveform Graph":ext[][])
    n79 = call "PeakDetector_Vector.vi"("threshold"=0.1, "FWD cut length"=10, "Variable_Num"=w69, "Signal Mode"=w75, "Input signal"=w38) -> ("Out signal"=w56:dbl[])  [unwired: 5 in, 1 out]
    n80 = Array Size(array=w56) -> (size(s)=w68:i32)
    n81 = for {
      N: w68 -> [_]
      tunnel: [w307] -> w64 mode=indexing
      tunnel: w61 -> [w307]
    }
    n82 = Divide(x=w33, y=w32) -> (x/y=w34:ext)
    n83 = Build Array (concatenate)(w66, w64) -> (w63:ext[])
    n84 = Build Array (concatenate)(w67, w56) -> (w62:ext[])
    n85 = Bundle(w63, w62) -> (→"Bifurcation Diagram":cluster{ext[], ext[]})  [unwired: 1 in]
    n86 = call "Bif_anal.vi"("n"=32.0, "Treshold"=0.01, "X"=w56) -> ("Y"=w70:dbl)  [unwired: 7 in, 1 out]
    n87 = call "Bif_anal_KDE.vi"("n"=32.0, "Manual h"=0.008 ("Treshold"), "X"=w56) -> ("Y"=w55:dbl)  [unwired: 7 in, 1 out]
  }
  n88 = Bundle(w6, w15) -> (w14:cluster{ext[], dbl[]})  [unwired: 1 in]
  n89 = Bundle(w6, w12) -> (w11:cluster{ext[], dbl[]})  [unwired: 1 in]
  n90 = Bundle(w6, w7) -> (w4:cluster{ext[], ext[]})  [unwired: 1 in]
  n91 = Bundle(w6, w5) -> (w3:cluster{ext[], dbl[]})  [unwired: 1 in]
  n92 = Build Array(w14, w11) -> (→"Mode Analysis":cluster{ext[], dbl[]}[])
  n93 = Build Array(w4, w3) -> (→"?":cluster{ext[], ext[]}[])
